vi "Exam.vi"() -> ()   [LabVIEW 2018]
uses:
  <vilib>/DAQmx/read.llb/DAQmx Read (Analog Wfm 1Chan NSamp).vi
  <vilib>/DAQmx/create/channels.llb/DAQmx Create Channel (AI-Voltage-Basic).vi
  <vilib>/DAQmx/configure/timing.llb/DAQmx Timing (Sample Clock).vi
  <vilib>/DAQmx/miscellaneous.llb/DAQmx Fill In Error Info.vi
panel:
  out "루프시간":u32
  out "실행횟수":i32
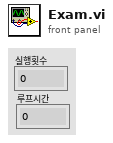
[diagram p1: front panel]
types:
  T1 = enum16{"open", "open or create", "create or replace", "create", "open (read-only)"}
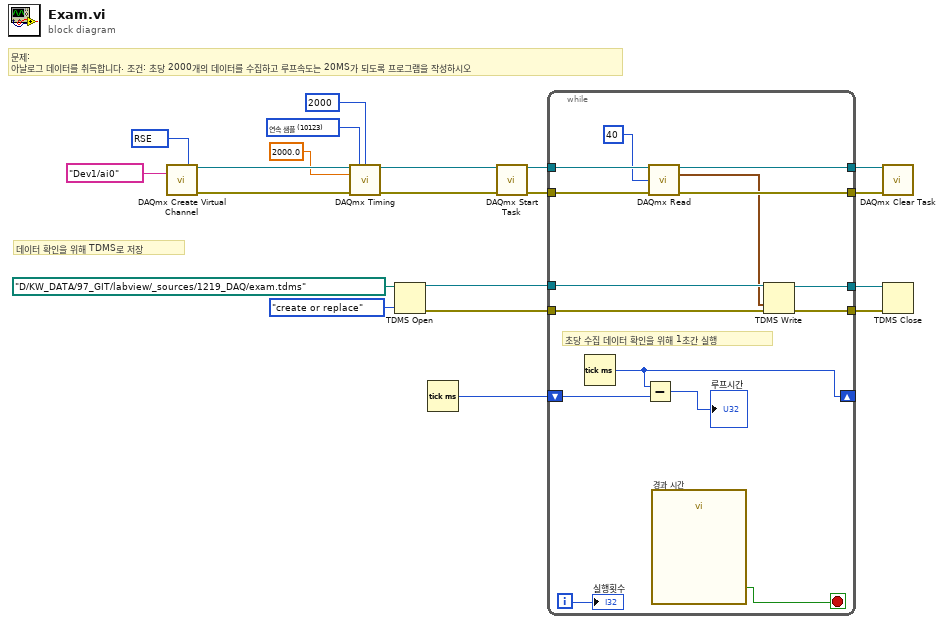
[diagram p0: block diagram]
diagram:
  w10 = 10123 items=["유한 샘플"=10178, "연속 샘플"=10123, "하드웨어 타이밍에 의한 단일 포인트"=12522] ("sample mode")
  w11 = 10083 items=["기본"=-1, "RSE"=10083, "NRSE"=10078, "차동"=10106, "유사 차동"=12529] ("input terminal configuration")
  # "데이터 확인을 위해 TDMS로 저장"
  # "문제: \n아날로그 데이터를 취득합니다. 조건: 초당 2000개의 데이터를 수집하고 루프속도는 20MS가 되도록 프로그램을 작성하시오"
  n1 = call-poly <vilib>:"DAQmx Create Virtual Channel.vi"("input terminal configuration"=w11, "physical channels"=tag "Dev1/ai0") -> ("task out"=w20:refnum<k21>, "error out"=w19:errorcluster)  [unwired: 12 in]
  n2 = call-poly <vilib>:"DAQmx Timing.vi"("task/channels in"=w20, "sample mode"=w10, "samples per channel"=2000, "rate"=2000.0, "error in"=w19) -> ("task out"=w18:refnum<k21>, "error out"=w17:errorcluster)  [unwired: 9 in]
  n3 = TDMS Open(10:T1."create or replace" ("동작(0:open)"), 11:path "D:/KW_DATA/97_GIT/labview/_sources/1219_DAQ/exam.tdms" ("파일 경로")) -> (0:w7:errorcluster, 3:w8:refnum<k34>)  [unwired: 5 in]
  n4 = Tick Count (ms)() -> (millisecond timer value=w1:u32)
  n5 = call <vilib>:"DAQmx Start Task.vi"("task/channels in"=w18, "error in"=w17) -> ("task out"=w16:refnum<k21>, "error out"=w15:errorcluster)  [unwired: 12 in]
  n6 = while {
    tunnel: w16 -> [w35]
    tunnel: w15 -> [w34]
    tunnel: [w33] -> w14
    tunnel: [w32] -> w13
    tunnel: w8 -> [w31]
    tunnel: w7 -> [w30]
    tunnel: [w29] -> w6
    tunnel: [w28] -> w5
    shift-right: [w22] -> _
    shift-left: w1 -> [w23]
    i -> [w25]
    stop <- w26 stop-if-true
    # "초당 수집 데이터 확인을 위해 1초간 실행"
    n7 = Tick Count (ms)() -> (millisecond timer value=w22:u32)
    n8 = Subtract(x=w22, y=w23) -> (x-y=→"루프시간":u32)
    n9 = call-poly <vilib>:"DAQmx Read.vi"("task/channels in"=w35, "number of samples per channel"=40, "error in"=w34) -> ("task out"=w33:refnum<k21>, "data"=w27:waveform(dbl), "error out"=w32:errorcluster)  [unwired: 10 in]
    n10 = call "경과 시간"() -> ("Time has Elapsed"=w26:bool)  [unwired: 12 in, 7 out]
    n11 = TDMS Write(0:w31, 9:w27, 11:w30) -> (4:w29:refnum<k34>, 15:w28:errorcluster)  [unwired: 3 in, 2 out]
    "실행횟수" <- w25
  }
  n12 = call <vilib>:"DAQmx Clear Task.vi"("task in"=w14, "error in"=w13) -> ()  [unwired: 13 in, 1 out]
  n13 = TDMS Close(8:w5, 11:w6) -> ()  [unwired: 2 out]
